vi "Connect.vi"(8 "error in (no error)":errorcluster, 11 "IP address":string="10.10.1.1") -> (0 "error out":errorcluster, 3 "connection ID":i32)   [LabVIEW 2009, in "MicroDAQ.lvlib"]
doc: "Connectes to microDAQ device via TCP/IP."
uses:
  <instrlib>/MicroDAQ/MicroDAQ.lvlib
  <instrlib>/MicroDAQ/Mlink library wraper/mlink.lvlib
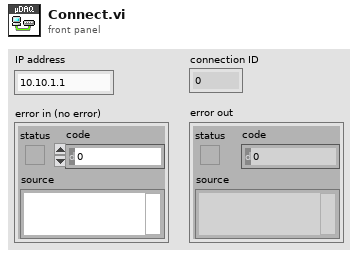
[diagram p1: front panel]
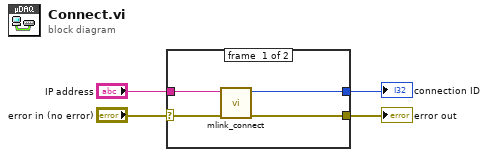
[diagram p0: block diagram]
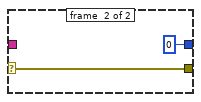
[diagram p2: hidden frame]
diagram:
  n1 = case shown="No Error" "error in (no error)" {
    selector: "error in (no error)" -> [w7 w9]
    tunnel: "IP address" -> [w8 _]
    tunnel: [w6 w9] -> w2
    tunnel: [w5 0 ("connection ID")] -> w1
    frame #0 {
      n2 = call <instrlib>:"mlink_connect.vi"("error in (no error)"=w7, "IP address"=w8) -> ("error out"=w6:errorcluster, "connection ID"=w5:i32)  [unwired: 8 in]
    }
    frame #1 {
    }
  }
  "error out" <- w2
  "connection ID" <- w1
